vi "Get Video Processor.vi"(2 "Camera?":bool, 3 "Video File":refnum<class "Video File.lvclass">) -> (0 "Video Processor":refnum<class "Video Processor.lvclass">, 1 "Video Cam Processor":refnum<class "Video Cam Processor.lvclass">)   [LabVIEW 2018]
uses:
  Classes/Video File/Video File.lvclass
  Classes/Video Cam Processor/Video Cam Processor.lvclass
  Classes/Video Processor/Video Processor.lvclass
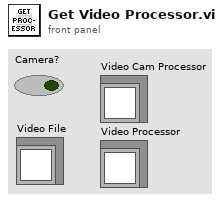
[diagram p1: front panel]
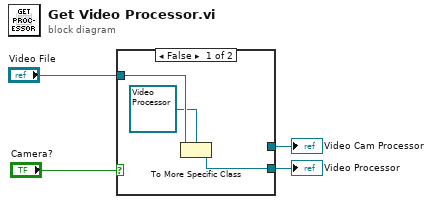
[diagram p0: block diagram]
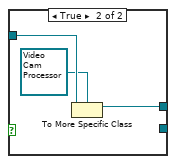
[diagram p2: hidden frame]
diagram:
  n1 = case shown="False" "Camera?" {
    tunnel: "Video File" -> [w7 w10]
    tunnel: [_ w8] -> w2
    tunnel: [w5 _] -> w1
    frame False {
      n2 = To More Specific Class(target class=refnum<class "Video Processor.lvclass"> refnum ("Video Processor.lvclass"), reference=w7) -> (specific class reference=w5:refnum<class "Video Processor.lvclass">)  [unwired: 1 in, 1 out]
    }
    frame True {
      n3 = To More Specific Class(target class=refnum<class "Video Cam Processor.lvclass"> refnum ("Video Cam Processor.lvclass"), reference=w10) -> (specific class reference=w8:refnum<class "Video Cam Processor.lvclass">)  [unwired: 1 in, 1 out]
    }
  }
  "Video Cam Processor" <- w2
  "Video Processor" <- w1
